vi "Get SMO Database Paths.vi"(5 "getAll Cluster":variant, 7 "Paths":string="llab_038:d000(TEST_TABLE--Temperature(Kelvin))\nllab_038:d002(TEST_TABLE--voltage 2(volts))\nllab_038:b000(TEST_TABLE--ON?())\nllab_038:v001(TEST_TABLE--sample())", 8 "error in (no error)":errorcluster, 11 "Inst.Xeryon-Rotator in":refnum<class "Inst.Xeryon-Rotator.lvclass">) -> (0 "error out":errorcluster, 2 "Paths":string, 3 "Inst.Xeryon-Rotator out":refnum<class "Inst.Xeryon-Rotator.lvclass">)   [LabVIEW 2019, in "Inst.Xeryon-Rotator.lvclass"]
uses:
  Inst.Xeryon-Rotator.lvclass
  Typedefs/Inst.Xeryon-Rotator.getAll--Cluster.ctl
  <userlib>/LevyLab/Instrument Framework/Instrument Types/Cryostat/Instrument.Cryostat.lvclass
  <userlib>/LevyLab/LV-Data/LV-Data.PG/LV-Data.PGSQL.lvclass
  <userlib>/LevyLab/LV-Data/LV-Data.PG/API/Write Variable (one-row).vi
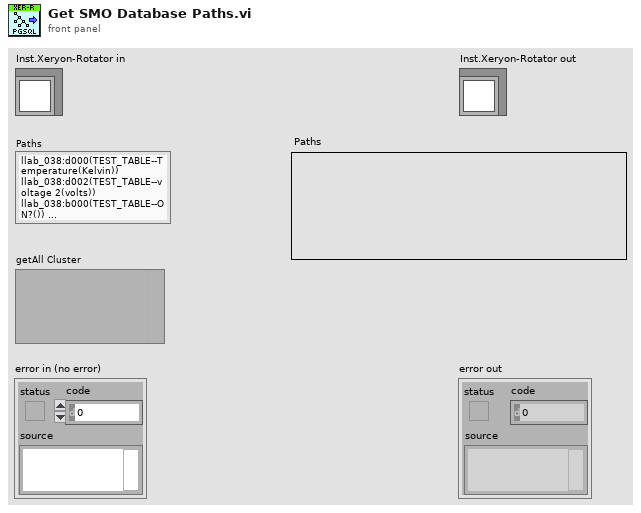
[diagram p1: front panel]
types:
  T1 = typedef "Inst.Xeryon-Rotator.lvclass/Inst.Xeryon-Rotator.getAll--Cluster.ctl" = cluster{"Encoder position [selected units]":dbl, "Desired Position [selected units]":dbl, "Status":string, "SRNO":dbl, "SOFT":dbl, "STAT":dbl, "FREQ":dbl, "OFRQ":dbl, "CURR":dbl, "SYNC":dbl, "Encoder Position [enc. units]":dbl, "Desired Position [enc. units]":dbl, "TIME":dbl, "Index Found":bool, "Left Limit":bool, "Right Limit":bool, "Position Reached":bool}
  T2 = cluster{"Encoder position [selected units]":dbl, "Desired Position [selected units]":dbl, "Status":string}
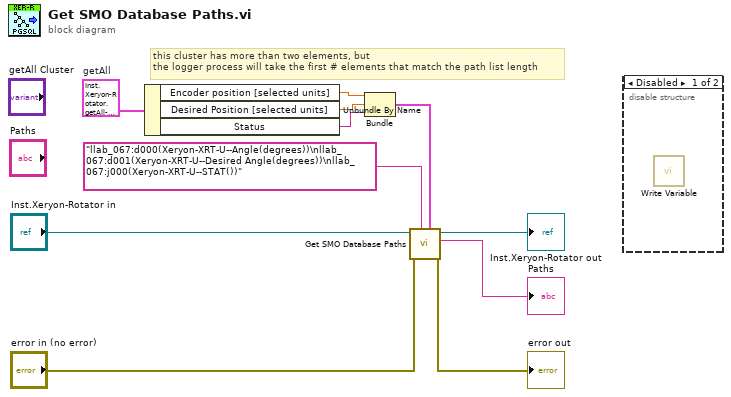
[diagram p0: block diagram]
diagram:
  w5 = T1 {"Encoder position [selected units]"=0.0, "Desired Position [selected units]"=0.0, "Status"="", "SRNO"=0.0, "SOFT"=0.0, "STAT"=0.0, "FREQ"=0.0, "OFRQ"=0.0, "CURR"=0.0, "SYNC"=0.0, "Encoder Position [enc. units]"=0.0, "Desired Position [enc. units]"=0.0, "TIME"=0.0, "Index Found"=FALSE, "Left Limit"=FALSE, "Right Limit"=FALSE, "Position Reached"=FALSE}  # getAll
  # "this cluster has more than two elements, but\nthe logger process will take the first # elements that match the path list length"
  n1 = Unbundle By Name(w5) -> ("Encoder position [selected units]"=w4:dbl, "Desired Position [selected units]"=w3:dbl, "Status"=w1:string)
  n2 = Bundle("Encoder position [selected units]"=w4, "Desired Position [selected units]"=w3, "Status"=w1) -> (w2:T2)  [unwired: 1 in]
  n3 = call-parent "Get SMO Database Paths.vi"("getAll Cluster"=w2, "Default Paths"="llab_067:d000(Xeryon-XRT-U--Angle(degrees))\nllab_067:d001(Xeryon-XRT-U--Desired Angle(degrees))\nllab_067:j000(Xeryon-XRT-U--STAT())" ("Paths"), "error in (no error)"="error in (no error)", "Instrument in"="Inst.Xeryon-Rotator in") -> ("error out"=→"error out":errorcluster, "Paths"=→"Paths":string, "Instrument out"=→"Inst.Xeryon-Rotator out":refnum<class "Inst.Xeryon-Rotator.lvclass">)  [unwired: 5 in]
  n4 = disable-structure shown="Disabled" {
    frame Disabled {
      n5 = call-poly <userlib>:"Write Variable.vi"() -> ()  [unwired: 8 in, 4 out]
    }
    frame Enabled {
    }
  }
